vi "Convert SEPL Parameters.vi"(0 "Phasor Parameters":T1={"Display Parameters"={"# Points"=0, "Ramp Type"=enum."Linear", "Type of Series"=enum."1-Exp Decays", "Min tau"=0.0, "Max tau"=0.0, "Include 0"=FALSE, "Include Infinity"=FALSE}, "Phasor Parameters"={"Harmonic Frequency"=0.0, "Use f* = 1/D Frequency"=FALSE, "Calibrated Phasor"=FALSE, "Calibration Lifetime"=1e-09, "Phasor Calculation"=enum."Direct Sum", "SEPL Type"=enum."UC", "# Gates"=1.0, "Square Gate Width"=1e-09, "Show Ticks"=FALSE}, "Decay & IRF Parameters"={"Lifetime"=0.0, "IRF Offset"=0.0, "IRF Period"=0.0, "Normalized Decays"=FALSE, "IRF Model"=enum."Dirac", "IRF Parameter 1"=0.0}, "Gate Parameters"={"First Gate Start"=0.0, "Use Gate Center"=FALSE, "Gate Width"=0.0, "Gate Step"=0.0, "# Gates"=0.0, "Gate Type"=enum."Square", "Edge Width"=0.0, "Top Slope"=0.0, "Reversed Sawtooth?"=FALSE, "Analytical Computation"=FALSE, "Integration"=enum."Item 0", "Tolerance"=1.0, "# Steps"=1.0, "Type of User-defined Function"=enum."Gate", "Use Gate Step"=FALSE}, "Detector Parameters"={"Frames/Image"=0, "Gates/Frame"=0, "Bits/Frame"=0, "Multiplicity"=0, "Incident Signal"=0.0, "Poisson Signal"=FALSE}} {"Detector Parameters"."Frames/Image" min=1; "Detector Parameters"."Multiplicity" min=0; "Detector Parameters"."Bits/Frame" min=1; "Detector Parameters"."Gates/Frame" min=1; "Gate Parameters"."# Steps" min=0.0; "Gate Parameters"."Tolerance" min=0.0; "Gate Parameters"."Top Slope" min=0.0; "Gate Parameters"."Edge Width" min=0.0; "Gate Parameters"."Gate Step" min=0.0; "Gate Parameters"."# Gates" min=0.0 step=1.0; "Gate Parameters"."Gate Width" min=0.0; "Decay & IRF Parameters"."Lifetime" min=0.0; "Decay & IRF Parameters"."IRF Period" min=0.0; "Phasor Parameters"."Square Gate Width" min=0.0; "Phasor Parameters"."# Gates" min=0.0; "Phasor Parameters"."Calibration Lifetime" min=0.0; "Phasor Parameters"."Harmonic Frequency" min=0.0; "Display Parameters"."Min tau" min=0.0; "Display Parameters"."Max tau" min=0.0; "Display Parameters"."# Points" min=1 step=1}, 9 "Linear Coefficients":cluster{"u":dbl, "v":dbl}, 11 "Error In":errorcluster) -> (4 "Ramp Type":enum16{"Linear", "Logarithmic"}(ring), 6 "Min tau":dbl, 8 "Max tau":dbl, 10 "# Steps":i32, 14 "Data for Pseudo UC Intersections":T13={"Linear Coefficients"={"u"=0.0, "v"=0.0}, "Decay Definition"={"offset: t0"=0.0, "period: T"=0.0, "lifetime: tau"=0.0, "Incident Signal: I"=0.5, "Normalized Decays"=FALSE, "IRF Model"=enum."Dirac", "IRF Parameter 1"=0.0, "Poisson Signal"=FALSE}, "Gates Definitions"={"First Gate: t1"=0.0, "Gate Width: W"=0.0, "Gate Step: d"=0.0, "# Gates: G"=0.0, "Use Gate Center"=FALSE, "Frames/Image: F"=50, "Gates/Frame: L"=0, "Bits/Frame: q"=0, "Multiplicity: p"=0, "Gate Type"=enum."Square", "Gate Edge s"=4.0, "Gate Top Slope"=4.0, "Reversed Sawtooth?"=FALSE, "Computation"=FALSE, "User-defined Gate"={"X Array"=[], "Y Array"=[]}, "Tolerance"=50.0, "Integration"=enum."Item 0", "# Steps"=50.0, "Type of User-defined Function"=enum."Gate"}, "iw"=0.0+0.0i, "Phasor Calculation"=enum."Direct Sum"}, 15 "Error Out":errorcluster)   [LabVIEW 2019]
uses:
  Data for SEPL Intersections.ctl
  Decay Definiton.ctl
  IRF Model.ctl
  Gate Definitions.ctl
  Gate Type.ctl
  Graphs/XY Graph/XY Plot Data.ctl
  Phasor Calculation Type.ctl
  SEPL Parameters.ctl
  Phasor Explorer Display Parameters.ctl
  Type of Series.ctl
  Phasor Explorer Phasor Parameters.ctl
  SEPL Type.ctl
  Phasor Explorer Decay Parameters.ctl
  Phasor Explorer Gate Parameters.ctl
  Type of User-defined Function.ctl
  Phasor Explorer Detector Parameters.ctl
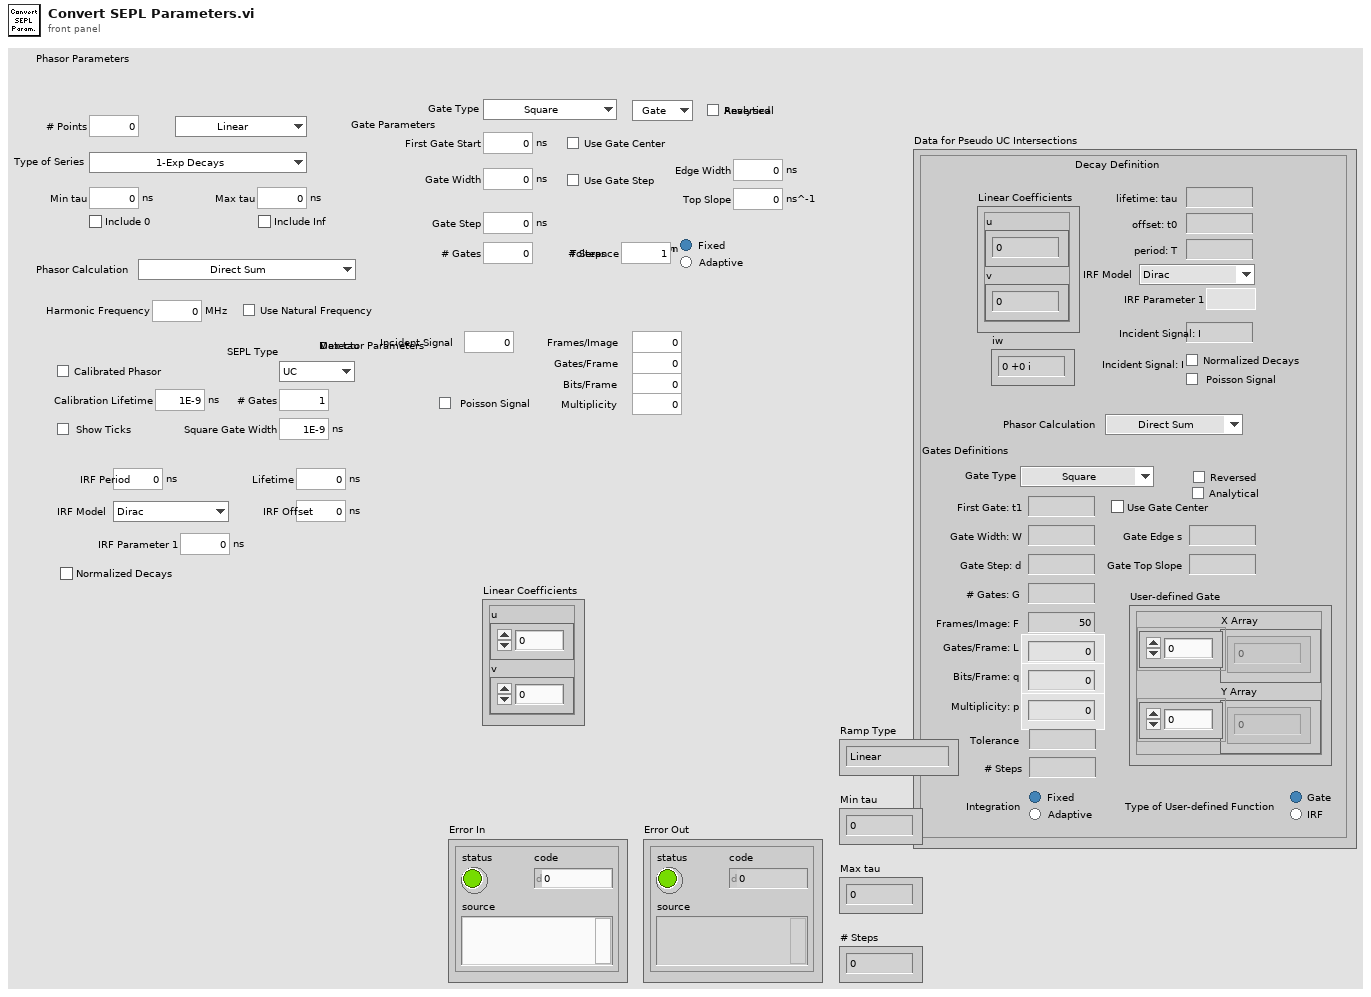
[diagram p1: front panel]
types:
  T1 = typedef "SEPL Parameters.ctl" = cluster{"Display Parameters":T2, "Phasor Parameters":T4, "Decay & IRF Parameters":T7, "Gate Parameters":T9, "Detector Parameters":T12}
  T2 = typedef "Phasor Explorer Display Parameters.ctl" = cluster{"# Points":i32, "Ramp Type":enum16{"Linear", "Logarithmic"}, "Type of Series":T3, "Min tau":dbl[unit], "Max tau":dbl[unit], "Include 0":bool, "Include Infinity":bool}
  T3 = typedef "Type of Series.ctl" = enum16{"1-Exp Decays", "Linear Combination of 1-Exp"}
  T4 = typedef "Phasor Explorer Phasor Parameters.ctl" = cluster{"Harmonic Frequency":dbl[unit], "Use f* = 1/D Frequency":bool, "Calibrated Phasor":bool, "Calibration Lifetime":dbl[unit], "Phasor Calculation":T5, "SEPL Type":T6, "# Gates":dbl, "Square Gate Width":dbl[unit], "Show Ticks":bool}
  T5 = typedef "Phasor Calculation Type.ctl" = enum16{"Direct Sum", "Analytical Formula"}
  T6 = typedef "SEPL Type.ctl" = enum16{"UC", "L_N", "L_N[W]", "L_X"}
  T7 = typedef "Phasor Explorer Decay Parameters.ctl" = cluster{"Lifetime":dbl[unit], "IRF Offset":dbl[unit], "IRF Period":dbl[unit], "Normalized Decays":bool, "IRF Model":T8, "IRF Parameter 1":dbl[unit]}
  T8 = typedef "IRF Model.ctl" = enum16{"Dirac", "Exponential"}
  T9 = typedef "Phasor Explorer Gate Parameters.ctl" = cluster{"First Gate Start":dbl[unit], "Use Gate Center":bool, "Gate Width":dbl[unit], "Gate Step":dbl[unit], "# Gates":dbl, "Gate Type":T10, "Edge Width":dbl[unit], "Top Slope":dbl[unit], "Reversed Sawtooth?":bool, "Analytical Computation":bool, "Integration":enum32{"Item 0", "Item 1"}, "Tolerance":dbl, "# Steps":dbl, "Type of User-defined Function":T11, "Use Gate Step":bool}
  T10 = typedef "Gate Type.ctl" = enum16{"Square", "Finite Edge Square", "Finite Edge, Tilted Top Square", "Triangle", "Sawtooth", "User-defined"}
  T11 = typedef "Type of User-defined Function.ctl" = enum16{"Gate", "IRF"}
  T12 = typedef "Phasor Explorer Detector Parameters.ctl" = cluster{"Frames/Image":i32, "Gates/Frame":i32, "Bits/Frame":i32, "Multiplicity":i32, "Incident Signal":dbl, "Poisson Signal":bool}
  T13 = typedef "Data for SEPL Intersections.ctl" = cluster{"Linear Coefficients":cluster{"u":dbl, "v":dbl}, "Decay Definition":T14, "Gates Definitions":T15, "iw":cdb, "Phasor Calculation":T5}
  T14 = typedef "Decay Definiton.ctl" = cluster{"offset: t0":ext, "period: T":ext, "lifetime: tau":ext, "Incident Signal: I":ext, "Normalized Decays":bool, "IRF Model":T8, "IRF Parameter 1":ext, "Poisson Signal":bool}
  T15 = typedef "Gate Definitions.ctl" = cluster{"First Gate: t1":ext, "Gate Width: W":ext, "Gate Step: d":ext, "# Gates: G":ext, "Use Gate Center":bool, "Frames/Image: F":i32, "Gates/Frame: L":i32, "Bits/Frame: q":i32, "Multiplicity: p":i32, "Gate Type":T10, "Gate Edge s":ext, "Gate Top Slope":ext, "Reversed Sawtooth?":bool, "Computation":bool, "User-defined Gate":T16, "Tolerance":ext, "Integration":enum32{"Item 0", "Item 1"}, "# Steps":ext, "Type of User-defined Function":enum32{"Gate", "IRF"}}
  T16 = typedef "XY Plot Data.ctl" = cluster{"X Array":dbl[], "Y Array":dbl[]}
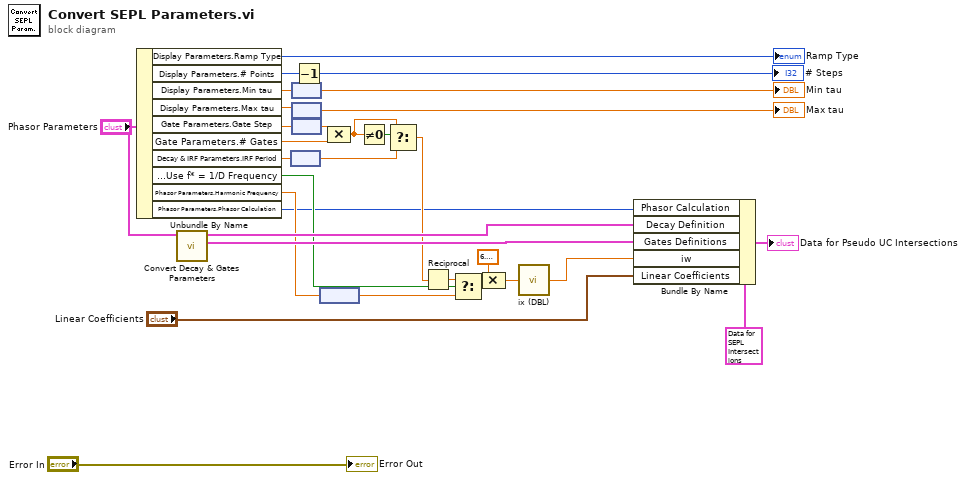
[diagram p0: block diagram]
diagram:
  n1 = Unbundle By Name("Phasor Parameters") -> ("Display Parameters.Ramp Type"=→"Ramp Type":enum16{"Linear", "Logarithmic"}, "Display Parameters.# Points"=w27:i32, "Display Parameters.Min tau"=w19:dbl[unit], "Display Parameters.Max tau"=w15:dbl[unit], "Gate Parameters.Gate Step"=w22:dbl[unit], "Gate Parameters.# Gates"=w23:dbl, "Decay & IRF Parameters.IRF Period"=w5:dbl[unit], "Phasor Parameters.Use f* = 1/D Frequency"=w10:bool, "Phasor Parameters.Harmonic Frequency"=w9:dbl[unit], "Phasor Parameters.Phasor Calculation"=w2:T5)
  n2 = call "Convert Decay & Gates Parameters.vi"("Phasor Parameters"="Phasor Parameters") -> ("Gates Definitions"=w11:T15, "Decay Definition"=w12:T14)  [unwired: 9 in]
  n3 = node(w5) -> (w3:dbl)
  n4 = node(w19) -> (→"Min tau":dbl)
  n5 = node(w15) -> (→"Max tau":dbl)
  n6 = node(w22) -> (w24:dbl)
  n7 = Decrement(x=w27) -> (x-1=→"# Steps":i32)
  n8 = node(w9) -> (w17:dbl)
  n9 = Compound Arithmetic op=MULTIPLY(w24, w23) -> (w6:dbl)
  n10 = Not Equal To 0?(x=w6) -> (x != 0?=w7:bool)
  n11 = Select(t=w6, s=w7, f=w3) -> (s? t:f=w4:dbl)
  n12 = Reciprocal(x=w4) -> (1/x=w8:dbl)
  n13 = Select(t=w8, s=w10, f=w17) -> (s? t:f=w18:dbl)
  n14 = Compound Arithmetic op=MULTIPLY(6.283185307179586, w18) -> (w1:dbl)
  n15 = call "ix (DBL).vi"("x (1)"=w1) -> ("i.(x)"=w28:cdb)
  n16 = Bundle By Name(cluster=T13 {"Linear Coefficients"={"u"=0.0, "v"=0.0}, "Decay Definition"={"offset: t0"=0.0, "period: T"=0.0, "lifetime: tau"=0.0, "Incident Signal: I"=0.5, "Normalized Decays"=FALSE, "IRF Model"=enum."Dirac", "IRF Parameter 1"=0.0, "Poisson Signal"=FALSE}, "Gates Definitions"={"First Gate: t1"=0.0, "Gate Width: W"=0.0, "Gate Step: d"=0.0, "# Gates: G"=0.0, "Use Gate Center"=FALSE, "Frames/Image: F"=50, "Gates/Frame: L"=0, "Bits/Frame: q"=0, "Multiplicity: p"=0, "Gate Type"=enum."Square", "Gate Edge s"=4.0, "Gate Top Slope"=4.0, "Reversed Sawtooth?"=FALSE, "Computation"=FALSE, "User-defined Gate"={"X Array"=[], "Y Array"=[]}, "Tolerance"=50.0, "Integration"=enum."Item 0", "# Steps"=50.0, "Type of User-defined Function"=enum."Gate"}, "iw"=0.0+0.0i, "Phasor Calculation"=enum."Direct Sum"}, "Phasor Calculation"=w2, "Decay Definition"=w12, "Gates Definitions"=w11, "iw"=w28, "Linear Coefficients"="Linear Coefficients") -> (→"Data for Pseudo UC Intersections":T13)
  "Error Out" <- "Error In"
